vi "commandMoveHardpointActuators.vi"(8 "error in (no error)":errorcluster, 10 "CommandMoveHardpointActuators in":T1, 11 "M1M3SAL in":refnum<class "M1M3SAL.lvclass">) -> (0 "error out":errorcluster, 2 "CommandMoveHardpointActuators out":T1, 3 "M1M3SAL out":refnum<class "M1M3SAL.lvclass">)   [LabVIEW 2016, in "M1M3SupportCommunicator.lvlib" / "M1M3SAL.lvclass"]
uses:
  M1M3SAL.lvclass
  DataTypes/Topics/CommandMoveHardpointActuators.ctl
  DataTypes/Topics/Parts/CommandId.ctl
  DataTypes/MessageHeader.ctl
  DataTypes/MessageTypes.ctl
  DataTypes/MessageTopics.ctl
  M1M3SAL.lvclass/M1M3SAL.ctl
  writeU8.vi
  writeI32.vi
  writeI8.vi
  M1M3SupportCommunicator.lvlib
  DataTypes/Topics/M1M3SupportTopics.lvlib
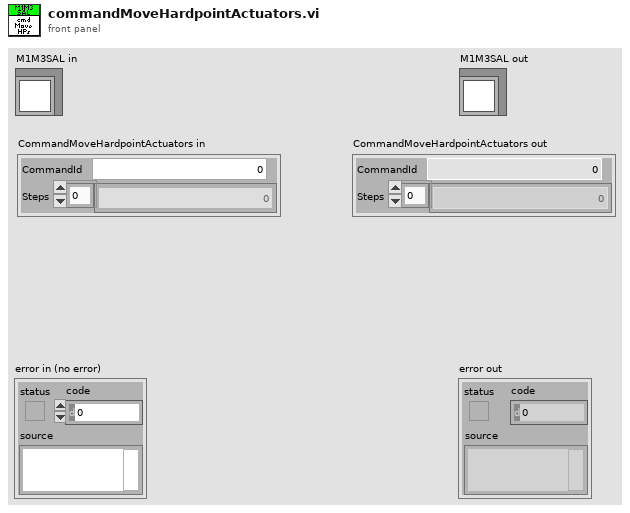
[diagram p1: front panel]
types:
  T1 = typedef "M1M3SupportTopics.lvlib/CommandMoveHardpointActuators.ctl" = cluster{"CommandId":T2, "Steps":i8[]}
  T2 = typedef "M1M3SupportTopics.lvlib/CommandId.ctl" = i32
  T3 = typedef "M1M3SupportCommunicator.lvlib/MessageHeader.ctl" = cluster{"Type":T4, "Topic":T5, "Size":i32}
  T4 = typedef "M1M3SupportCommunicator.lvlib/MessageTypes.ctl" = enum8{"None", "PutSample", "GetNextSample", "LogEvent", "GetEvent", "IssueCommand", "CommandId", "WaitForCompletion", "AcceptCommand", "AckCommand"}
  T5 = typedef "M1M3SupportCommunicator.lvlib/MessageTopics.ctl" = enum8{"None", "ForceActuatorData", "MirrorForceData", "HardpointData", "AirData", "DynamicData", "FPGAData", "IMSData", "ForceActuatorStatus", "ElevationData", "HardpointStatus", "HardpointActuatorChase", "AirStatus", "ForceActuatorSafetyChecks", "ForceActuatorTest", "ActuatorBroadcastCounter", "StatusChecks", "CellChecks", "HardpointActuatorBreakaway", "RaiseMirrorComplete", "ILCCommunication", "ElevationAngleChecks", "DetailedState", "ServoLoops", "ForceActuatorInfo", "LowerMirrorComplete", "HardpointActuatorInfo", "SettingsApplied", "ErrorCode", "StartupChecks", "SummaryState", "SettingVersions", "ActuatorTestStatus", "AppliedSettingsMatchStart", "Enable", "EnterMaintenance", "Standby", "AbortLowerM1M3", "ApplyAberrationByForces", "ApplyAOSCorrectionByBendingModes", "ClearAOSCorrection", "Start", "RaiseM1M3", "TestForceActuator", "LowerM1M3", "ApplyAOSCorrectionByForces", "Disable", "ApplyAberationByBendingMode", "TestHardpoint", "ManipulateM1M3", "ClearAberration", "Exit", "TestAir", "AbortRaiseM1M3", "MoveHardpointActuators", "ExitMaintenance", "Shutdown"}
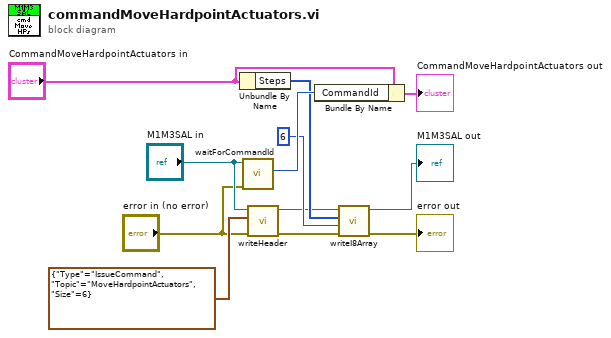
[diagram p0: block diagram]
diagram:
  n1 = Unbundle By Name("CommandMoveHardpointActuators in") -> ("Steps"=w7:i8[])
  n2 = call "waitForCommandId.vi"("error in (no error)"="error in (no error)", "M1M3SAL in"="M1M3SAL in") -> ("CommandId"=w11:T2)  [unwired: 7 in, 2 out]
  n3 = call "writeHeader.vi"("error in (no error)"="error in (no error)", "MessageHeader"=T3 {"Type"=enum."IssueCommand", "Topic"=enum."MoveHardpointActuators", "Size"=6}, "M1M3SAL in"="M1M3SAL in") -> ("error out"=w4:errorcluster, "M1M3SAL out"=w2:refnum<class "M1M3SAL.lvclass">)  [unwired: 7 in]
  n4 = Bundle By Name(cluster="CommandMoveHardpointActuators in", "CommandId"=w11) -> (→"CommandMoveHardpointActuators out":T1)
  n5 = call "writeI8Array.vi"("error in (no error)"=w4, "Length"=6, "Input"=w7, "M1M3SAL in"=w2) -> ("error out"=→"error out":errorcluster, "M1M3SAL out"=→"M1M3SAL out":refnum<class "M1M3SAL.lvclass">)  [unwired: 6 in]
